vi "add_int32.vi"   [LabVIEW 2014]
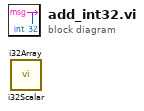
[diagram p0: block diagram]
diagram:
  n1 = call "i32Scalar.vi"() -> ()  [unwired: 5 in, 1 out]
  n2 = call "i32Array.vi"() -> ()  [unwired: 5 in, 1 out]
